vi "Build Plots.vi"(10 "Listbox":i32[](array[numeric]), 11 "Event Data Array in":dbl[][](array[numeric])) -> (2 "Labels":string[](array[string]), 3 "Sensor Plots":dynamicdata(graph))   [LabVIEW 2021]
uses:
  <vilib>/express/express shared/transition.llb/Dynamic To Waveform Array.vi
  <vilib>/express/express signal manip/GetorSetDDTAttributes/Set DDT Attributes/SetT0.vi
  <vilib>/express/express shared/transition.llb/Waveform Array To Dynamic.vi
  <vilib>/express/express signal manip/GetorSetDDTAttributes/Set DDT Attributes/Set DDT Properties.xnode
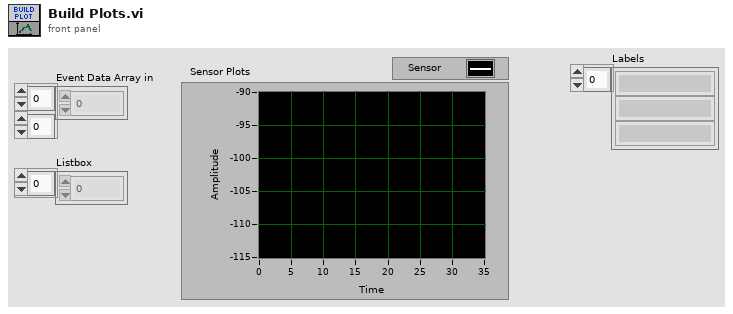
[diagram p1: front panel]
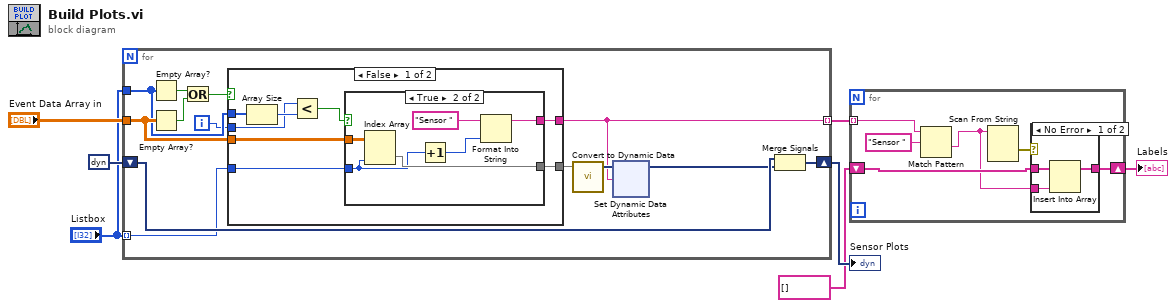
[diagram p0: block diagram]
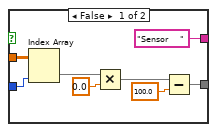
[diagram p3: hidden frame]
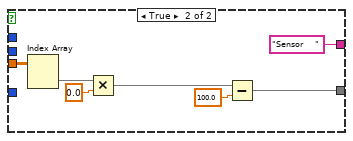
[diagram p4: hidden frame]
diagram:
  n1 = for {
    tunnel: "Event Data Array in" -> [w20]
    tunnel: "Listbox" -> [w19]
    shift-right: [w10] -> w5
    shift-left: dynamicdata [] ("Waveform Graph 2") -> [w12]
    tunnel: [w9] -> w3 mode=indexing
    tunnel: "Listbox" -> [w8] mode=indexing
    i -> [w15]
    n2 = Empty Array?(array=w19) -> (empty?=w17:bool)
    n3 = Empty Array?(array=w20) -> (empty?=w16:bool)
    n4 = Or(x=w17, y=w16) -> (x .or. y?=w18:bool)
    n5 = case shown="False" w18 {
      tunnel: [w36 w58] -> w14
      tunnel: w20 -> [w37 w59]
      tunnel: w19 -> [w42 _]
      tunnel: [w41 "Sensor    "] -> w9
      tunnel: w15 -> [w38 _]
      tunnel: w8 -> [w35 _]
      frame False {
        n6 = Array Size(array=w42) -> (size(s)=w39:i32)
        n7 = Less?(x=w38, y=w39) -> (x < y?=w40:bool)
        n8 = case shown="True" w40 {
          tunnel: ["Sensor    " w55] -> w41
          tunnel: w37 -> [w49 w54]
          tunnel: w35 -> [w48 w52]
          tunnel: [w43 w53] -> w36
          frame False {
            n9 = Index Array(array=w49, index (col)=w48) -> (element=w47:dbl[])  [unwired: 1 in]
            n10 = Multiply(x=w47, y=0.0) -> (x*y=w45:dbl[])
            n11 = Subtract(x=w45, y=100.0) -> (x-y=w43:dbl[])
          }
          frame True {
            n12 = Index Array(array=w54, index (col)=w52) -> (element=w53:dbl[])  [unwired: 1 in]
            n13 = Increment(x=w52) -> (x+1=w51:i32)
            n14 = Format Into String(initial string="Sensor ", w51) -> (resulting string=w55:string)  [unwired: 2 in, 1 out]
          }
        }
      }
      frame True {
        n15 = Index Array(array=w59) -> (element=w62:dbl[])  [unwired: 2 in]
        n16 = Multiply(x=w62, y=0.0) -> (x*y=w61:dbl[])
        n17 = Subtract(x=w61, y=100.0) -> (x-y=w58:dbl[])
      }
    }
    n18 = call "Convert to Dynamic Data"("Array"=w14) -> ("Dynamic Data Type"=w13:dynamicdata)  [unwired: 3 in]
    n19 = xnode "Set Dynamic Data Attributes"("Signals In"=w13, "Signal Name"=w9) -> ("Signals Out"=w11:dynamicdata)  [unwired: 2 in, 1 out]
    n20 = Merge Signals(w12, w11) -> (w10:dynamicdata)
  }
  "Sensor Plots" <- w5
  n21 = for {
    tunnel: w3 -> [w66] mode=indexing
    shift-right: [w68] -> w2
    shift-left: string[] [] -> [w69]
    n22 = Match Pattern(string=w66, regular expression="Sensor ") -> (after substring=w64:string)  [unwired: 1 in, 3 out]
    n23 = Scan From String(input string=w64) -> (error out=w67:errorcluster)  [unwired: 5 in, 2 out]
    n24 = case shown="No Error" w67 {
      tunnel: w69 -> [w72 w73]
      tunnel: w64 -> [w70 _]
      tunnel: [w71 w73] -> w68
      frame No Error {
        n25 = Insert Into Array(array=w72, new element=w70) -> (w71:string[])  [unwired: 1 in]
      }
      frame Error {
      }
    }
  }
  "Labels" <- w2
